vi "TCP-error.vi"   [LabVIEW 2013, in "HardwareCharacterization.lvlib" / "HC-SM1000.lvclass"]
uses:
  HC-SM1000.lvclass
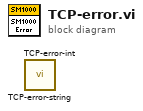
[diagram p0: block diagram]
diagram:
  n1 = call "TCP-error-string.vi"() -> ()  [unwired: 11 in, 1 out]
  n2 = call "TCP-error-int.vi"() -> ()  [unwired: 11 in, 1 out]
